vi "In Range Array.vi"(1 "Array":dbl[](array[numeric]), 2 "lower limit":dbl, 3 "upper limit":dbl=15.0) -> (0 "At least 1 out of range":bool)   [LabVIEW 2011]
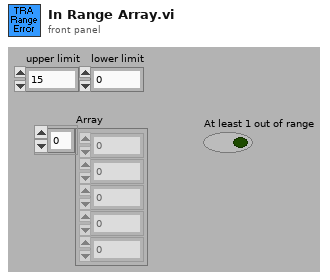
[diagram p1: front panel]
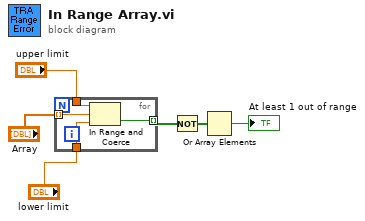
[diagram p0: block diagram]
diagram:
  n1 = for {
    tunnel: "Array" -> [w10] mode=indexing
    tunnel: [w9] -> w4 mode=indexing
    tunnel: "upper limit" -> [w8]
    tunnel: "lower limit" -> [w7]
    n2 = In Range and Coerce(upper limit=w8, x=w10, lower limit=w7) -> (In Range?=w9:bool)  [unwired: 1 out]
  }
  n3 = Not(x=w4) -> (.not. x?=w5:bool[])
  n4 = Or Array Elements(Boolean array=w5) -> (logical OR=→"At least 1 out of range":bool)
